vi "Createrollrefcsv.vi"() -> ()   [LabVIEW 2019]
uses:
  <vilib>/LabVIEW Open Source Project/Data Manipulation/Scalar/FinalStringFormatting.vi
  <vilib>/LabVIEW Open Source Project/Data Manipulation/Scalar/Get Decimal Separator.vi
  <vilib>/Utility/file.llb/Write Delimited Spreadsheet (string).vi
  <vilib>/LabVIEW Open Source Project/Data Manipulation/Scalar/OpenScalar.lvlib
panel:
  in  "Time step":dbl
  in  "Rollref":dbl
  out "timestep":dbl
  out "rollreff":dbl
  in  "stop":bool
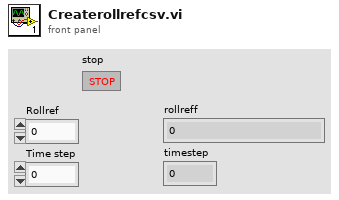
[diagram p1: front panel]
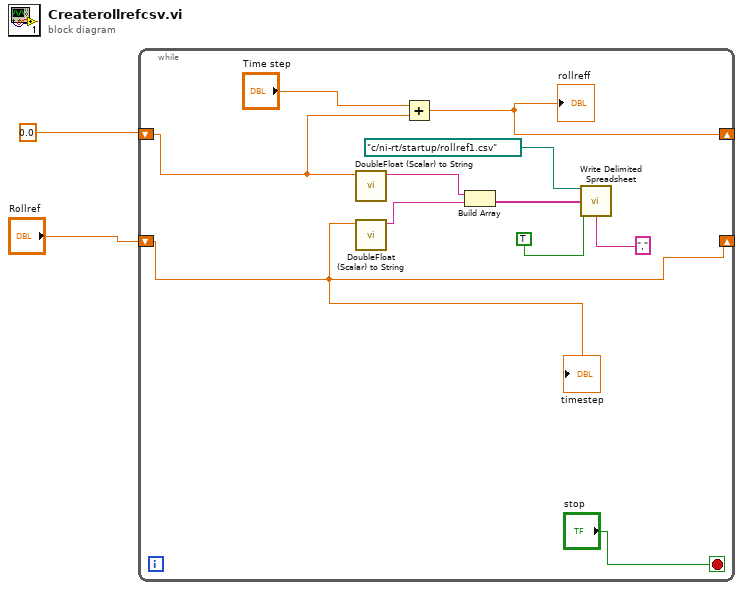
[diagram p0: block diagram]
diagram:
  n1 = while {
    shift-right: [w4] -> _
    shift-left: 0.0 -> [w5]
    shift-right: [w6] -> _
    shift-left: "Rollref" -> [w6]
    stop <- "stop" stop-if-true
    n2 = call <vilib>:"DoubleFloat (Scalar) to String.vi"("Value (Double)"=w5) -> ("Value (String)"=w12:string)  [unwired: 10 in]
    n3 = call <vilib>:"DoubleFloat (Scalar) to String.vi"("Value (Double)"=w6) -> ("Value (String)"=w11:string)  [unwired: 10 in]
    n4 = Add(x="Time step", y=w5) -> (x+y=w4:dbl)
    "rollreff" <- w4
    n5 = Build Array(w12, w11) -> (w8:string[])
    n6 = call-poly <vilib>:"Write Delimited Spreadsheet.vi"("file path (dialog if empty)"=path "c:/ni-rt/startup/rollref1.csv", "1D data"=w8, "append to file? (new file:F)"=TRUE, "delimiter (\\t)"="," ("delimiter (\\t)")) -> ()  [unwired: 10 in, 2 out]
    "timestep" <- w6
  }
